vi "当时日期.vi"(11 "待处理日期":string) -> (1 "年份":i32, 2 "月":i32, 3 "日":i32)   [LabVIEW 2018]
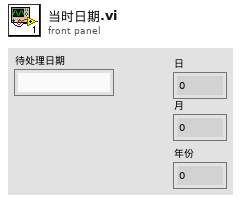
[diagram p1: front panel]
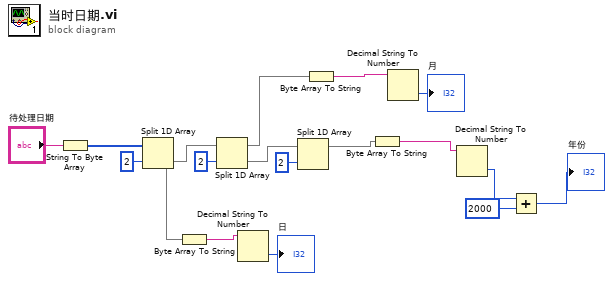
[diagram p0: block diagram]
diagram:
  n1 = String To Byte Array(string="待处理日期") -> (unsigned byte array=w17:u8[])
  n2 = Split 1D Array(array=w17, index=2 ("索引")) -> (first subarray=w10:u8[], second subarray=w16:u8[])
  n3 = Byte Array To String(unsigned byte array=w10) -> (string=w8:string)
  n4 = Split 1D Array(array=w16, index=2 ("索引")) -> (first subarray=w9:u8[], second subarray=w15:u8[])
  n5 = Decimal String To Number(string=w8) -> (number=→"日":i32)  [unwired: 2 in, 1 out]
  n6 = Split 1D Array(array=w15, index=2 ("索引")) -> (first subarray=w14:u8[])  [unwired: 1 out]
  n7 = Byte Array To String(unsigned byte array=w9) -> (string=w7:string)
  n8 = Byte Array To String(unsigned byte array=w14) -> (string=w6:string)
  n9 = Decimal String To Number(string=w7) -> (number=→"月":i32)  [unwired: 2 in, 1 out]
  n10 = Decimal String To Number(string=w6) -> (number=w3:i32)  [unwired: 2 in, 1 out]
  n11 = Add(x=w3, y=2000) -> (x+y=→"年份":i32)
